vi "Parse SmartCOM Message 2.vi"(0 "Message":string, 1 "Delimiter [/ ]":string="[/ ]", 3 "Names":string[](array[string])) -> (8 "From Alias":string, 10 "From Alias Index":i32=-1, 12 "Message Subclass":string, 14 "Root Message":string, 15 "Param 1":string, 16 "Param 2":string, 17 "All Params":string[](array[string]), 18 "Message Class":string, 19 "Message Exists":bool)   [LabVIEW 2023]
uses:
  <vilib>/Utility/error.llb/Trim Whitespace One-Sided.vi
  <vilib>/regexp/Match Regular Expression.xnode
panel:
  out "regex":string
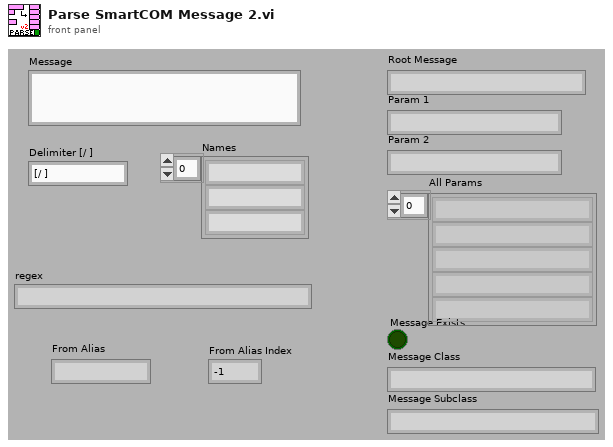
[diagram p1: front panel]
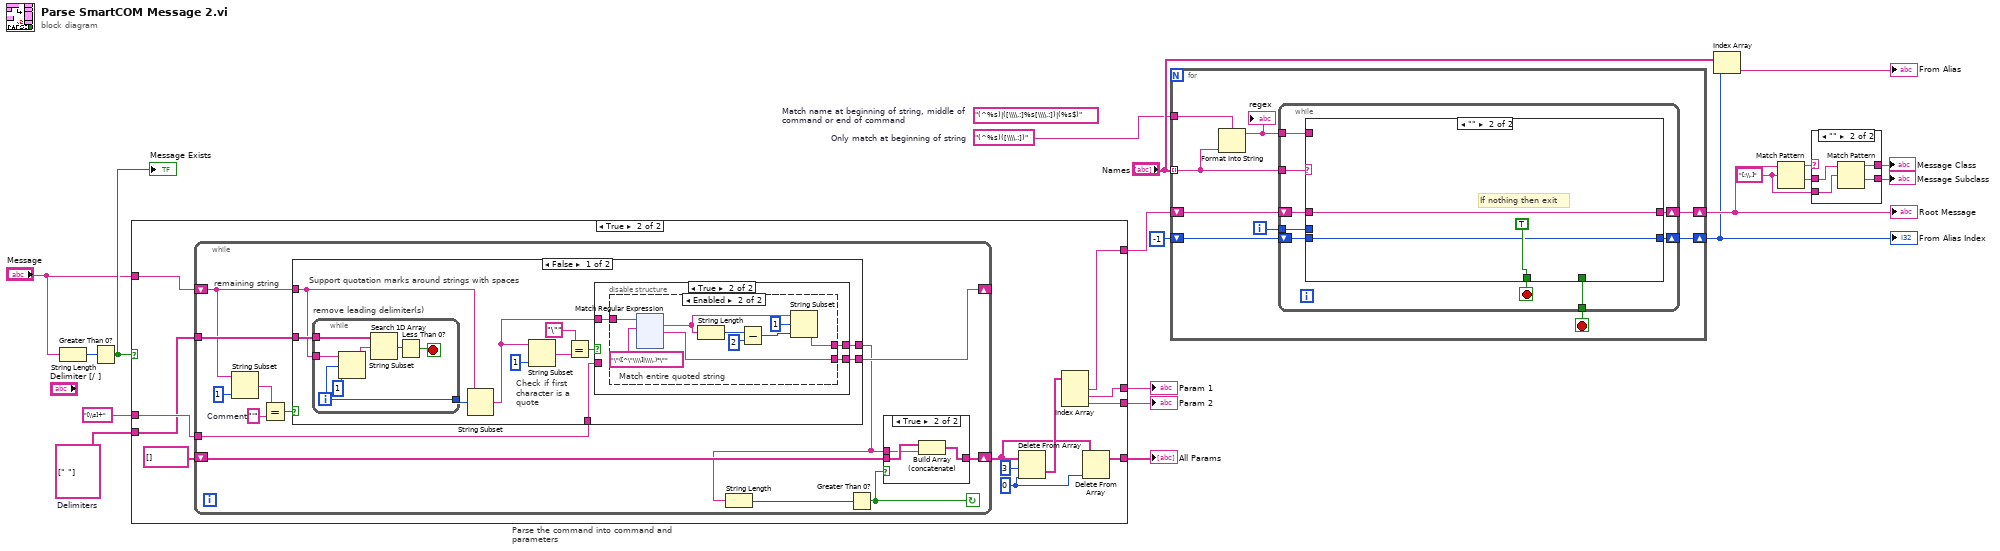
[diagram p0: block diagram]
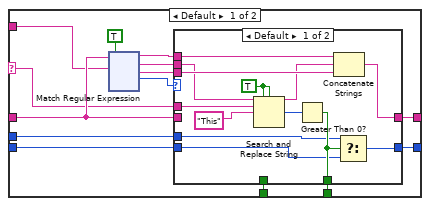
[diagram p2: hidden frame]
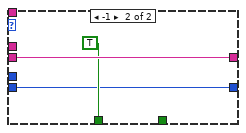
[diagram p3: hidden frame]
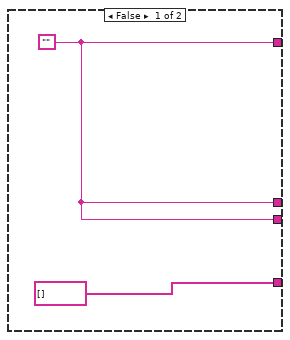
[diagram p5: hidden frame]
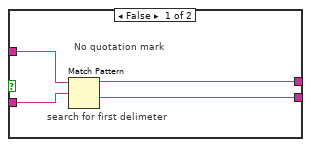
[diagram p6: hidden frame]
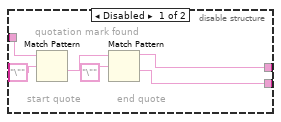
[diagram p7: hidden frame]
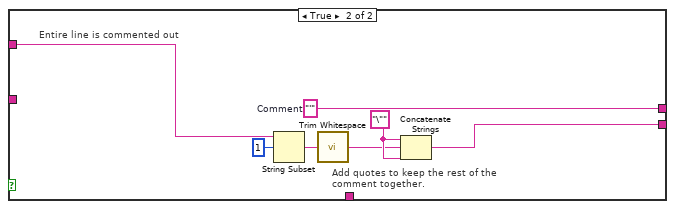
[diagram p8: hidden frame]
diagram:
  w1 = "(^%s)([\\\\.:])"  # Only match at beginning of string
  (unwired) "(^%s)|([\\\\.:]%s[\\\\.:])|(%s$)"  # Match name at beginning of string, middle of command or end of command
  w10 = "[:\\.]" ("regular expression")
  w13 = string[] [" "]  # Delimiters
  n1 = String Length(string="Message") -> (length=w20:i32)
  n2 = Greater Than 0?(x=w20) -> (x > 0?=w19:bool)
  "Message Exists" <- w19
  n3 = case shown="True" w19 {
    tunnel: "Message" -> [_ w32]
    tunnel: "[\\s]+" ("Delimiter [/ ]") -> [_ w34]
    tunnel: [w22 w31] -> w8
    tunnel: [w22 w23] -> w18
    tunnel: [w22 w30] -> w17
    tunnel: [string[] [] ("Params") w25] -> w16
    tunnel: w13 -> [_ w27]
    frame False {
      w22 = ""
    }
    frame True {
      w24 = 0 ("index")
      n4 = while "Parse the command into command and parameters" {
        shift-right: [w43] -> _
        shift-left: w32 -> [w40]
        tunnel: w34 -> [w42]
        shift-right: [w45] -> w26
        shift-left: string[] [] ("Params") -> [w46]
        tunnel: w27 -> [w41]
        stop <- w44 continue-if-true
        w37 = "'"  # Comment
        # "remaining string"
        n5 = String Subset(string=w40, length (rest)=1 ("length (rest)")) -> (substring=w38:string)  [unwired: 1 out]
        n6 = Equal?(x=w38, y=w37) -> (x = y?=w36:bool)
        n7 = case shown="False" w36 {
          tunnel: [w58 w211] -> w35
          tunnel: [w57 w207] -> w43
          tunnel: w42 -> [w56 _]
          tunnel: w41 -> [w54 _]
          tunnel: w40 -> [w48 w210]
          frame False {
            # "Support quotation marks around strings with spaces"
            # "Check if first character is a quote"
            n8 = while "remove leading delimiter(s)" {
              tunnel: w54 -> [w64]
              tunnel: [w60] -> w55
              tunnel: w48 -> [w59]
              i -> [w60]
              stop <- w61 stop-if-true
              n9 = String Subset(string=w59, offset (0)=w60, length (rest)=1 ("length (rest)")) -> (substring=w63:string)
              n10 = Search 1D Array(1D array=w64, element=w63) -> (index of element=w62:i32)  [unwired: 1 out]
              n11 = Less Than 0?(x=w62) -> (x < 0?=w61:bool)
            }
            n12 = String Subset(string=w48, offset (0)=w55) -> (substring=w49:string)  [unwired: 1 out]
            n13 = String Subset(string=w49, length (rest)=1 ("length (rest)")) -> (substring=w52:string)  [unwired: 1 out]
            n14 = Equal?(x="\"" ("regular expression"), y=w52) -> (x = y?=w50:bool)
            n15 = case shown="True" w50 {
              tunnel: w49 -> [w69 w72]
              tunnel: w56 -> [w68 _]
              tunnel: [w67 w71] -> w58
              tunnel: [w66 w70] -> w57
              frame False {
                # "search for first delimeter"
                # "No quotation mark"
                n16 = Match Pattern(string=w69, regular expression=w68) -> (before substring=w67:string, after substring=w66:string)  [unwired: 3 out]
              }
              frame True {
                n17 = disable-structure shown="Enabled" {
                  disable-tunnel: w72 -> [w78 w87]
                  disable-tunnel: [w76 w85] -> w71
                  disable-tunnel: [w75 w80] -> w70
                  frame Disabled {
                    # "end quote"
                    # "start quote"
                    # "quotation mark found"
                    n18 = Match Pattern(string=w78, regular expression="\"") -> (after substring=w77:string)  [unwired: 4 out]
                    n19 = Match Pattern(string=w77, regular expression="\"") -> (before substring=w76:string, after substring=w75:string)  [unwired: 3 out]
                  }
                  frame Enabled {
                    # "Match entire quoted string"
                    n20 = xnode "Match Regular Expression"("input string"=w87, "regular expression"="\"([^\"\\\\]|\\\\.)*\"") -> ("whole match"=w79:string, "after match"=w80:string)  [unwired: 2 in, 5 out]
                    n21 = String Length(string=w79) -> (length=w83:i32)
                    n22 = Subtract(x=w83, y=2 ("offset (0)")) -> (x-y=w81:i32)
                    n23 = String Subset(string=w79, offset (0)=1, length (rest)=w81) -> (substring=w85:string)
                  }
                }
              }
            }
          }
          frame True {
            w208 = "\""
            w211 = "'"  # Comment
            # "Add quotes to keep the rest of the comment together."
            # "Entire line is commented out"
            n24 = String Subset(string=w210, offset (0)=1) -> (substring=w206:string)  [unwired: 1 out]
            n25 = call <vilib>:"Trim Whitespace.vi"("string"=w206) -> ("trimmed string"=w205:string)  [unwired: 1 in]
            n26 = Concatenate Strings(w208, w205, w208) -> (w207:string)
          }
        }
        n27 = String Length(string=w35) -> (length=w47:i32)
        n28 = Greater Than 0?(x=w47) -> (x > 0?=w44:bool)
        n29 = case shown="True" w44 {
          tunnel: w46 -> [w212 w215]
          tunnel: [w212 w213] -> w45
          tunnel: w35 -> [_ w214]
          frame False {
          }
          frame True {
            n30 = Build Array (concatenate)(w215, w214) -> (w213:string[])
          }
        }
      }
      n31 = Delete From Array(array=w26, length=3, index=w24) -> (deleted portion=w28:string[])  [unwired: 1 out]
      n32 = Index Array(array=w28) -> (element #1=w31:string, element #2=w23:string, element #3=w30:string)  [unwired: 3 in]
      n33 = Delete From Array(array=w26, index=w24) -> (array with subset deleted=w25:string[])  [unwired: 1 in, 1 out]
    }
  }
  "Param 1" <- w18
  "Param 2" <- w17
  "All Params" <- w16
  n34 = for {
    tunnel: "Names" -> [w223] mode=indexing
    tunnel: w1 -> [w222]
    shift-right: [w220] -> w6
    shift-left: w8 -> [w224]
    shift-right: [w217] -> w2
    shift-left: -1 ("index") -> [w219]
    i -> [w218]
    stop <- w216 stop-if-true
    n35 = Format Into String(format string=w222, w223) -> (resulting string=w221:string)  [unwired: 2 in, 1 out]
    "regex" <- w221
    n36 = while {
      tunnel: w223 -> [w231]
      tunnel: w221 -> [w230]
      shift-right: [w232] -> w220
      shift-left: w224 -> [w233]
      tunnel: w218 -> [w227]
      tunnel: [w225] -> w216
      shift-right: [w226] -> w217
      shift-left: w219 -> [w228]
      stop <- w229 stop-if-true
      n37 = case shown="\"\"" w231 {
        selector: w231 -> [w240 _]
        tunnel: [w247 w383] -> w232
        tunnel: w233 -> [w242 w383]
        tunnel: w230 -> [w241 _]
        tunnel: [w238 TRUE] -> w229
        tunnel: w228 -> [w237 w381]
        tunnel: w227 -> [w236 _]
        tunnel: [w235 w381] -> w226
        tunnel: [w234 _] -> w225
        frame Default {
          n38 = xnode "Match Regular Expression"("input string"=w242, "regular expression"=w241, "ignore case? (F)"=TRUE ("replace all? (F)")) -> ("before match"=w246:string, "whole match"=w245:string, "after match"=w244:string, "offset past match"=w243:i32)  [unwired: 2 in, 2 out]
          n39 = case shown="Default" w243 {
            tunnel: [w375 w380] -> w247
            tunnel: w242 -> [_ w380]
            tunnel: w246 -> [w377 _]
            tunnel: w245 -> [w374 _]
            tunnel: w244 -> [w376 _]
            tunnel: w240 -> [w373 _]
            tunnel: [_ TRUE] -> w238
            tunnel: w237 -> [w365 w378]
            tunnel: w236 -> [w366 _]
            tunnel: [w368 w378] -> w235
            tunnel: [w367 _] -> w234
            frame Default {
              w370 = TRUE ("replace all? (F)")
              n40 = Search and Replace String(replace all?=w370, case sensitive?=w370, input string=w374, search string=w373, replace string="This" ("regular expression")) -> (result string=w371:string, number of replacements=w369:i32)  [unwired: 1 in, 4 out]
              n41 = Greater Than 0?(x=w369) -> (x > 0?=w367:bool)
              n42 = Concatenate Strings(w377, w371, w376) -> (w375:string)
              n43 = Select(t=w366, s=w367, f=w365) -> (s? t:f=w368:i32)
            }
            frame -1 {
            }
          }
        }
        frame "" {
          # "If nothing then exit"
        }
      }
    }
  }
  "Root Message" <- w6
  "From Alias Index" <- w2
  n44 = Index Array(array="Names", index=w2) -> (element=→"From Alias":string)
  n45 = Match Pattern(string=w6, regular expression=w10) -> (before substring=w7:string, after substring=w12:string)  [unwired: 3 out]
  n46 = case shown="\"\"" w7 {
    selector: w7 -> [w385 _]
    tunnel: w12 -> [w384 w389]
    tunnel: [w385 w388] -> w11
    tunnel: w10 -> [_ w387]
    tunnel: [w384 w386] -> w9
    frame Default {
    }
    frame "" {
      n47 = Match Pattern(string=w389, regular expression=w387) -> (before substring=w388:string, after substring=w386:string)  [unwired: 3 out]
    }
  }
  "Message Class" <- w11
  "Message Subclass" <- w9
